vi "Configure ALC Search.vi"(0 "VISA resource name":refnum<visa-resource-name>, 1 "Enable Power Protection (F:Disable)":bool, 2 "Power Search Reference (0: Modulated)":u16(ring) items=["Modulated", "Fixed"], 5 "Power Search Mode (0: On)":u16(ring) items=["On", "Off", "Once"], 7 "Enable Span Power Search (T:Enable)":bool=TRUE, 9 "Span Type (0: Full)":u16(ring) items=["Full", "User"], 11 "error in (no error)":errorcluster, 12 "Span Start Frequency (1 MHz)":dbl=1000000.0, 13 "Span Stop Frequency (2 MHz)":dbl=2000000.0) -> (4 "VISA resource name out":refnum<visa-resource-name>, 15 "error out":errorcluster)   [LabVIEW 2011, in "Agilent PSG MXG Series.lvlib"]
doc: "Configures the internal power search and the span mode.\n\n<B>Notes:</B>\n(1) This VI is valid only when ALC is OFF."
uses:
  Agilent PSG MXG Series.lvlib
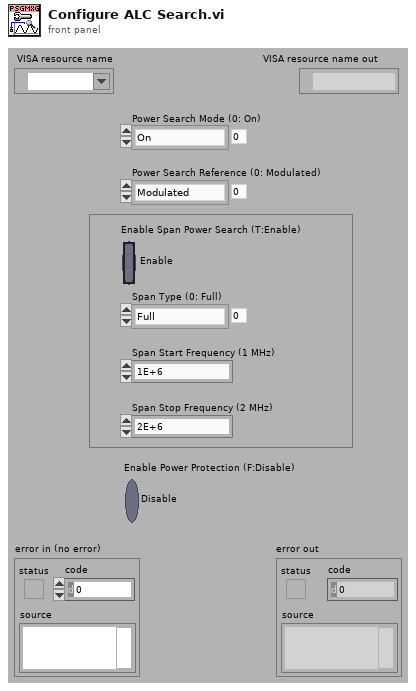
[diagram p1: front panel]
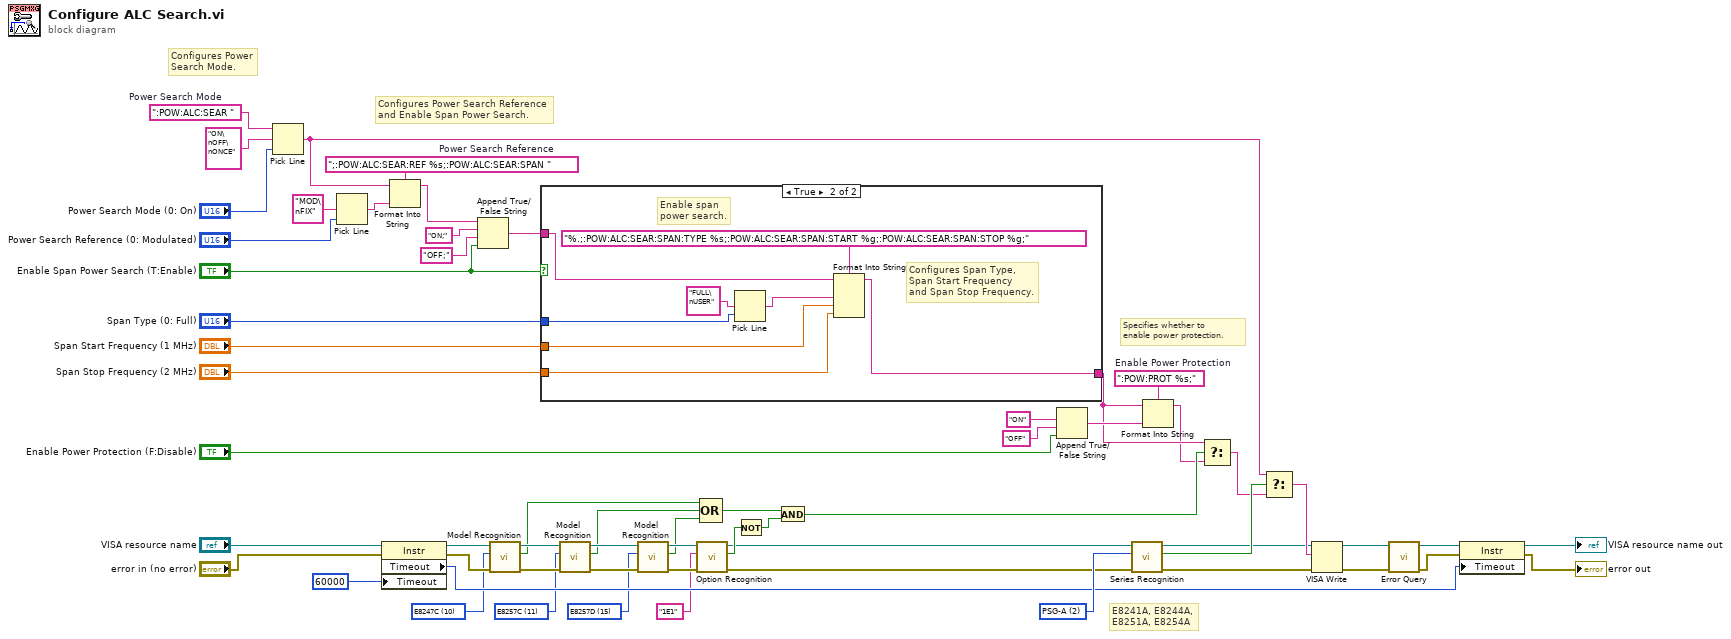
[diagram p0: block diagram]
diagram:
  w16 = u16 15 items=["N5181A"=0, "N5182A"=1, "N5183A"=2, "E8241A"=5, "E8244A"=6, "E8251A"=7, "E8254A"=8, "E8247C"=10, "E8257C"=11, "E8267C"=12, "E8257D"=15, "E8267D"=16] ("Model Type (0: N5181A)")
  w19 = u16 11 items=["N5181A"=0, "N5182A"=1, "N5183A"=2, "E8241A"=5, "E8244A"=6, "E8251A"=7, "E8254A"=8, "E8247C"=10, "E8257C"=11, "E8267C"=12, "E8257D"=15, "E8267D"=16] ("Model Type (0: N5181A)")
  w22 = u16 10 items=["N5181A"=0, "N5182A"=1, "N5183A"=2, "E8241A"=5, "E8244A"=6, "E8251A"=7, "E8254A"=8, "E8247C"=10, "E8257C"=11, "E8267C"=12, "E8257D"=15, "E8267D"=16] ("Model Type (0: N5181A)")
  w35 = u16 2 items=["MXG", "PSG", "PSG-A", "PSG-C", "PSG-D"] ("Series Type (0: MXG)")
  w45 = ":POW:PROT %s;"  # Enable Power Protection
  w57 = ";:POW:ALC:SEAR:REF %s;:POW:ALC:SEAR:SPAN "  # Power Search Reference
  w60 = ":POW:ALC:SEAR "  # Power Search Mode
  # "E8241A, E8244A,\nE8251A, E8254A"
  # "Specifies whether to\nenable power protection."
  # "Configures Power Search Reference\nand Enable Span Power Search."
  # "Configures Power\nSearch Mode."
  n1 = Pick Line(string ("")=w60, multi-line string="ON\nOFF\nONCE", line index="Power Search Mode (0: On)") -> (output string=w36:string)
  n2 = Pick Line(multi-line string="MOD\nFIX", line index="Power Search Reference (0: Modulated)") -> (output string=w56:string)  [unwired: 1 in]
  n3 = property class="Instr"(reference="VISA resource name", error in="error in (no error)", "Timeout"=u32 60000 ("General Settings:Timeout Value")) -> (reference out=w24:refnum<visa-resource-name>, error out=w23:errorcluster, "Timeout"=w27:u32)
  n4 = Format Into String(format string=w57, initial string=w36, w56) -> (resulting string=w53:string)  [unwired: 1 in, 1 out]
  n5 = Append True/False String(1:"Enable Span Power Search (T:Enable)", 2:"OFF;" ("false string"), 3:"ON;" ("true string"), 4:w53) -> (0:w49:string)
  n6 = call "Model Recognition.vi"("error in (no error)"=w23, "Model Type (0: N5181A)"=w22, "VISA resource name"=w24) -> ("error out"=w20:errorcluster, "Is Model Correct"=w12:bool, "VISA resource name out"=w21:refnum<visa-resource-name>)  [unwired: 6 in]
  n7 = case shown="True" "Enable Span Power Search (T:Enable)" {
    tunnel: w49 -> [w61 w69]
    tunnel: "Span Type (0: Full)" -> [_ w65]
    tunnel: "Span Start Frequency (1 MHz)" -> [_ w64]
    tunnel: "Span Stop Frequency (2 MHz)" -> [_ w63]
    tunnel: [w61 w62] -> w4
    frame False {
      # "Disable span power search."
    }
    frame True {
      # "Configures Span Type,\nSpan Start Frequency\nand Span Stop Frequency."
      # "Enable span\npower search."
      n8 = Pick Line(multi-line string="FULL\nUSER", line index=w65) -> (output string=w67:string)  [unwired: 1 in]
      n9 = Format Into String(format string="%.;:POW:ALC:SEAR:SPAN:TYPE %s;:POW:ALC:SEAR:SPAN:START %g;:POW:ALC:SEAR:SPAN:STOP %g;", initial string=w69, w67, w64, w63) -> (resulting string=w62:string)  [unwired: 1 in, 1 out]
    }
  }
  n10 = call "Model Recognition.vi"("error in (no error)"=w20, "Model Type (0: N5181A)"=w19, "VISA resource name"=w21) -> ("error out"=w17:errorcluster, "Is Model Correct"=w11:bool, "VISA resource name out"=w18:refnum<visa-resource-name>)  [unwired: 6 in]
  n11 = call "Model Recognition.vi"("error in (no error)"=w17, "Model Type (0: N5181A)"=w16, "VISA resource name"=w18) -> ("error out"=w14:errorcluster, "Is Model Correct"=w10:bool, "VISA resource name out"=w15:refnum<visa-resource-name>)  [unwired: 6 in]
  n12 = call "Option Recognition.vi"("error in (no error)"=w14, "Option (\"\")"="1E1" ("Option (\"\")"), "VISA resource name"=w15) -> ("error out"=w1:errorcluster, "Is Option Installed"=w9:bool, "VISA resource name out"=w2:refnum<visa-resource-name>)  [unwired: 6 in]
  n13 = Compound Arithmetic op=OR(w12, w11, w10) -> (w8:bool)
  n14 = Not(x=w9) -> (.not. x?=w7:bool)
  n15 = And(x=w8, y=w7) -> (x .and. y?=w5:bool)
  n16 = Append True/False String(1:"Enable Power Protection (F:Disable)", 2:"OFF" ("false string"), 3:"ON" ("true string")) -> (0:w44:string)  [unwired: 1 in]
  n17 = call "Series Recognition.vi"("error in (no error)"=w1, "Series Type (0: MXG)"=w35, "VISA resource name"=w2) -> ("error out"=w37:errorcluster, "Is Series Correct"=w39:bool, "VISA resource name out"=w38:refnum<visa-resource-name>)  [unwired: 6 in]
  n18 = Format Into String(format string=w45, initial string=w4, w44) -> (resulting string=w3:string)  [unwired: 1 in, 1 out]
  n19 = Select(t=w4, s=w5, f=w3) -> (s? t:f=w6:string)
  n20 = Select(t=w36, s=w39, f=w6) -> (s? t:f=w40:string)
  n21 = VISA Write(VISA resource name=w38, write buffer=w40, error in (no error)=w37) -> (VISA resource name out=w34:refnum<visa-resource-name>, error out=w33:errorcluster)  [unwired: 1 out]
  n22 = call "Error Query.vi"("error in (no error)"=w33, "VISA resource name"=w34) -> ("error out"=w28:errorcluster, "VISA resource name out"=w29:refnum<visa-resource-name>)  [unwired: 6 in, 2 out]
  n23 = property class="Instr"(reference=w29, error in=w28, "Timeout"=w27) -> (reference out=→"VISA resource name out":refnum<visa-resource-name>, error out=→"error out":errorcluster)
